vi "AuMT8852B EUT Address Source.vi"(5 "Source (Manual)":enum16{"Manual", "RS-232", "USB", "Inquiry"}(ring), 7 "Set/Get (Set)":enum16{"Set", "Get"}(ring), 8 "error in (no error)":errorcluster, 11 "VISA session":refnum<visa-resource-name>) -> (0 "error out":errorcluster, 2 "error code":i32, 3 "VISA session out":refnum<visa-resource-name>, 4 "Source out":enum16{"Manual", "RS-232", "USB", "Inquiry"}(ring))   [LabVIEW 2017]
doc: "Anritsu MT8852B Bluetooth Tester\n\nDetermines whether the EUT Bluetooth address will be set to a fixed value, queried over RS-232 / USB, or obtained through a Bluetooth inquiry.\n\nINPUTS\nSet/Get - whether the value is being sent to or retrieved from the instrument.\nSource - information to send to the instrument.\n\nOUTPUTS\nSource out - the present value in the instrument."
uses:
  <instrlib>/aumt8852B/General/Utilities/MT8850 Attribute ID.ctl
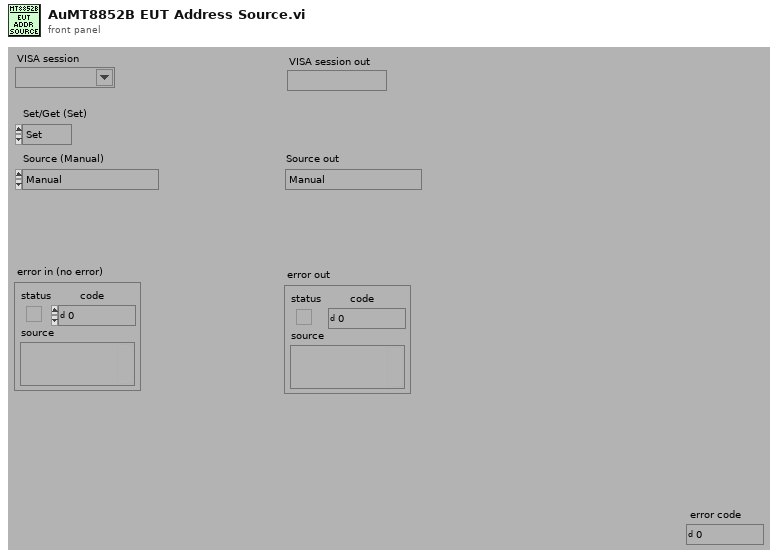
[diagram p1: front panel]
types:
  T1 = typedef "MT8850 Attribute ID.ctl" = enum16{"Operation mode", "Selected script", "EUT address source", "EUT Address", "EUT HCI RS232 Baud Rate", "Tester GPIB Address", "Tester RS232 Baud Rate", "Tester Bluetooth Address", "Tester Contrast", "Tester Key Click On", "Tester Modulation Index", "Tester Poll-Null Mode", "Tester Power Range", "Tester RS232 Mode", "Beep on Illegal Entry", "Display User Text", "User Text", "Calibration TX Modulation DAC", "Calibration RX Channel", "Calibration TX Channel", "Calibration TX Power", "Calibration Use TX Table", "Inquiry Request User-friendly Name", "Inquiry Number of Responses", "Inquiry Timeout", "Script Frequency Display", "Script Loop Count", "Script Loop Continuously", "Script Loop Stop on Fail", "Link timeout", "Page timeout", "Filter bandwidth", "SCO air code", "SCO bit position", "SCO input code", "SCO input data", "SCO input sample size", "SCO loopback mode", "SCO packet type", "SCO tone generator", "Tester page scan repetition mode", "Tester follow test mode", "Tester authentication state", "Tester authentication pin code", "Tester authentication pin length"}
  T2 = typedef "Attribute Status.ctl" = enum16{"No I/O needed", "I/O needed"}
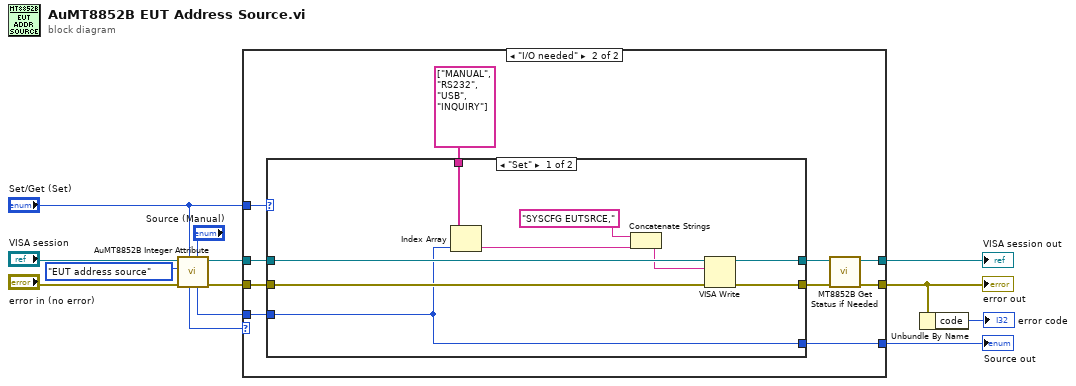
[diagram p0: block diagram]
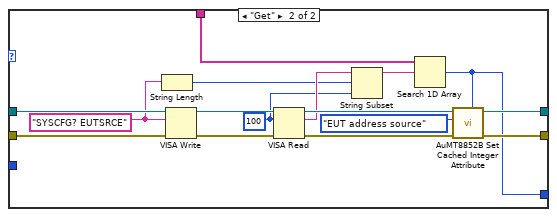
[diagram p3: hidden frame]
diagram:
  n1 = call <instrlib>:"AuMT8852B Integer Attribute.vi"("Value (0)"="Source (Manual)", "Set/Get (Set)"="Set/Get (Set)", "error in (no error)"="error in (no error)", "Attribute ID"=MT8850_Attribute_ID."EUT address source", "VISA session"="VISA session") -> ("error out"=w6:errorcluster, "VISA session out"=w7:refnum<visa-resource-name>, "Value out"=w9:i32, "Status"=w4:T2)  [unwired: 3 in]
  n2 = case shown="\"I/O needed\"" w4 {
    tunnel: "Set/Get (Set)" -> [_ w25]
    tunnel: w9 -> [w16 w24]
    tunnel: [w14 w17] -> w1
    tunnel: [w15 w18] -> w8
    tunnel: w7 -> [w15 w23]
    tunnel: w6 -> [w14 w22]
    tunnel: [w16 w21] -> w3
    frame "No I/O needed", Default {
    }
    frame "I/O needed" {
      n3 = case shown="\"Set\"" w25 {
        tunnel: [w27 w44] -> w19
        tunnel: string[] ["MANUAL", "RS232", "USB", "INQUIRY"] ("Array Constant") -> [w35 w40]
        tunnel: w24 -> [w32 _]
        tunnel: [w28 w45] -> w20
        tunnel: w23 -> [w34 w51]
        tunnel: w22 -> [w33 w50]
        tunnel: [w32 w43] -> w21
        frame "Set" {
          n4 = Index Array(array=w35, index=w32) -> (element=w30:string)
          n5 = Concatenate Strings("SYSCFG EUTSRCE," ("Substring"), w30) -> (w31:string)
          n6 = VISA Write(VISA resource name=w34, write buffer=w31, error in (no error)=w33) -> (VISA resource name out=w28:refnum<visa-resource-name>, error out=w27:errorcluster)  [unwired: 1 out]
        }
        frame "Get" {
          w38 = u32 100 ("byte count (0)")
          w37 = "SYSCFG? EUTSRCE" ("write buffer (\"\")")
          n7 = String Length(string=w37) -> (length=w36:i32)
          n8 = VISA Write(VISA resource name=w51, write buffer=w37, error in (no error)=w50) -> (VISA resource name out=w49:refnum<visa-resource-name>, error out=w48:errorcluster)  [unwired: 1 out]
          n9 = VISA Read(VISA resource name=w49, byte count=w38, error in (no error)=w48) -> (VISA resource name out=w47:refnum<visa-resource-name>, read buffer=w41:string, error out=w46:errorcluster)  [unwired: 1 out]
          n10 = String Subset(string=w41, offset (0)=w36, length (rest)=w38) -> (substring=w39:string)
          n11 = Search 1D Array(1D array=w40, element=w39) -> (index of element=w43:i32)  [unwired: 1 in]
          n12 = call <instrlib>:"AuMT8852B Set Cached Integer Attribute.vi"("Value (0)"=w43, "error in (no error)"=w46, "Attribute ID"=MT8850_Attribute_ID."EUT address source", "VISA session"=w47) -> ("error out"=w44:errorcluster, "VISA session out"=w45:refnum<visa-resource-name>)  [unwired: 6 in]
        }
      }
      n13 = call <instrlib>:"MT8852B Get Status if Needed.vi"("error in (no error)"=w19, "VISA session"=w20) -> ("error out"=w17:errorcluster, "VISA session out"=w18:refnum<visa-resource-name>)  [unwired: 8 in]
    }
  }
  "error out" <- w1
  "VISA session out" <- w8
  "Source out" <- w3
  n14 = Unbundle By Name(w1) -> ("code"=→"error code":i32)
